vi "test_HM_times_x_preload.vi"() -> ()   [LabVIEW 2017]
uses:
  fgm_pipiline_mine/x_vec_type.ctl
  quadProgControls/x_qp_scalar.ctl
  <vilib>/rvi/DesktopExecutionNode/Execution/niFpgaDEN_Execute.vi
  <vilib>/rvi/DesktopExecutionNode/DesktopExecutionNode.xnode
panel:
  out "x_vec":T1=[0.6000000238418579, 0.6000000238418579, -0.5999999940395355, -0.5999999940395355, 0.6000000238418579, 0.6000000238418579, 0.6000000238418579, 0.6000000238418579, -0.5999999940395355, 0.6000000238418579, -0.5999999940395355, -4.0, 0.0, 0.0, 0.0, 0.0, 0.0, 0.0, 0.0, 0.0, 0.0, 0.0, 0.0, 0.0, 0.0]
  out "A*x (expected, fp)":dbl[](array[numeric])
  out "A*x (expected, fxp)":fxp<+/-,32,3>[](array[numeric])
  in  "Ncol":u16
  in  "primary_write_addr":u16
  in  "preload_vec":fxp<+/-,32,3>[](array[numeric])=[0.0, 0.0, 0.0, 0.0, 0.0, 0.0, 0.0, 0.0, 0.0, 0.0, 0.0, 0.0]
  in  "preload_addr":u16
  in  "StartIndex":u16
  out "A*x":fxp<+/-,32,3>[](array[numeric])
  out "primary result":fxp<+/-,32,2>[](array[numeric])
  out "preload result":fxp<+/-,32,2>[](array[numeric])
  in  "SLMAX":fxp<+/-,18,5>
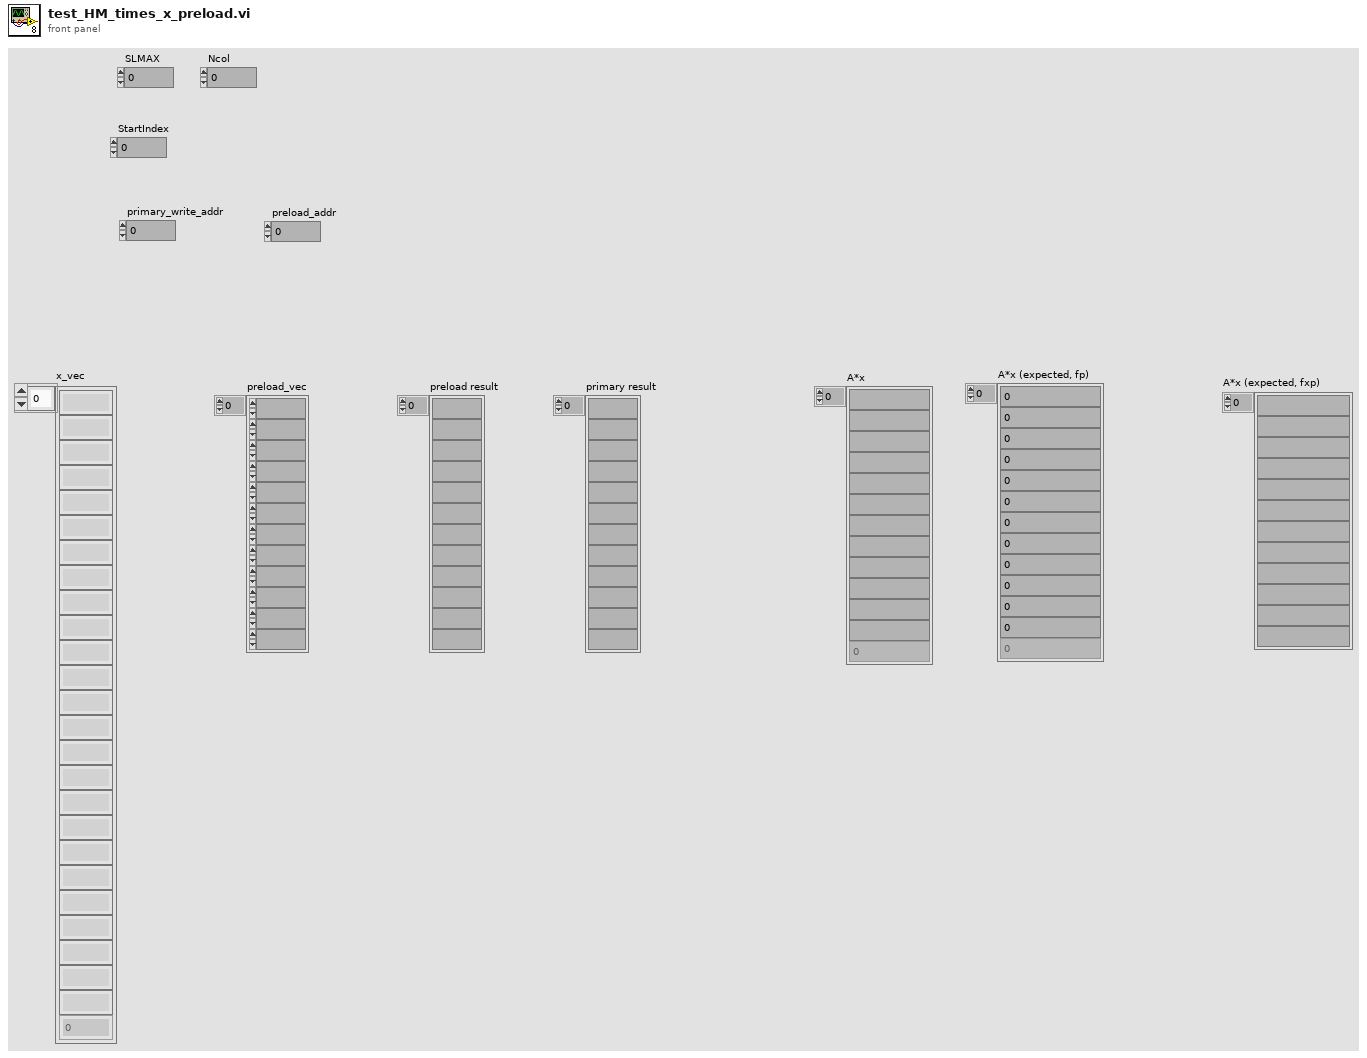
[diagram p1: front panel]
types:
  T1 = typedef "x_vec_type.ctl" = T2[]
  T2 = typedef "x_qp_scalar.ctl" = fxp<+/-,32,6>
  T3 = typedef "fgm_result_test_data.ctl" = cluster{"z_i_sequence":dbl[][], "y_i_sequence":dbl[][], "X_states":dbl[][]}
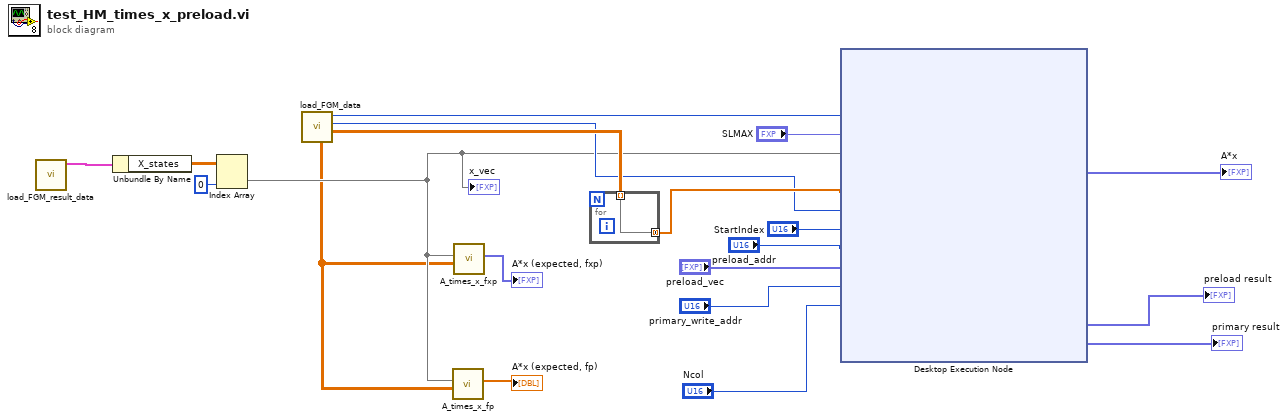
[diagram p0: block diagram]
diagram:
  n1 = call "load_FGM_result_data.vi"() -> ("FGM_result_data"=w5:T3)  [unwired: 10 in, 1 out]
  n2 = Unbundle By Name(w5) -> ("X_states"=w4:dbl[][])
  n3 = Index Array(array=w4, index (col)=0 ("disabled index (col)")) -> (element=w2:dbl[])  [unwired: 1 in]
  "x_vec" <- w2
  n4 = call "load_FGM_data.vi"() -> ("all rows"=w20:dbl[][], "Nmpc"=w10:i32, "Ns"=w17:i32, "M"=w1:dbl[][])  [unwired: 7 in, 1 out]
  n5 = call "A_times_x_fp.vi"("Az_mat in"=w1, "x_k"=w2) -> ("A*x"=→"A*x (expected, fp)":dbl[])  [unwired: 8 in, 1 out]
  n6 = call "A_times_x_fxp.vi"("Az_mat in"=w1, "x_k"=w2) -> ("A*x"=→"A*x (expected, fxp)":fxp<+/-,64,12>[])  [unwired: 8 in, 1 out]
  n7 = for {
    tunnel: w20 -> [w21] mode=indexing
    tunnel: [w21] -> w15 mode=concatenating
  }
  n8 = xnode "Desktop Execution Node"("Ns"=w17, "SLMAX"="SLMAX", "x_vec"=w2, "big_mat_data"=w15, "nuN_mpc"=w10, "StartIndex"="StartIndex", "preload_addr"="preload_addr", "preload_vec"="preload_vec", "primary_write_addr"="primary_write_addr", "Ncol"="Ncol") -> ("A*x"=→"A*x":fxp<+/-,32,3>[], "preload result"=→"preload result":fxp<+/-,32,2>[], "primary result"=→"primary result":fxp<+/-,32,2>[])  [unwired: 1 in, 1 out]
